vi "ConvertDesiredRefreshRatioPerReactor.vi"(0 "Desired Refresh Ratio":dbl, 2 "Reactor":i64 min=0 max=7) -> (1 "Required Number of Pump Iterations":dbl)   [LabVIEW 2016]
uses:
  CurrentSwitchValues_GlobalVariable.vi
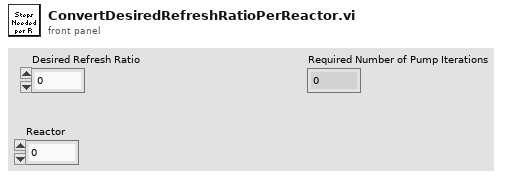
[diagram p1: front panel]
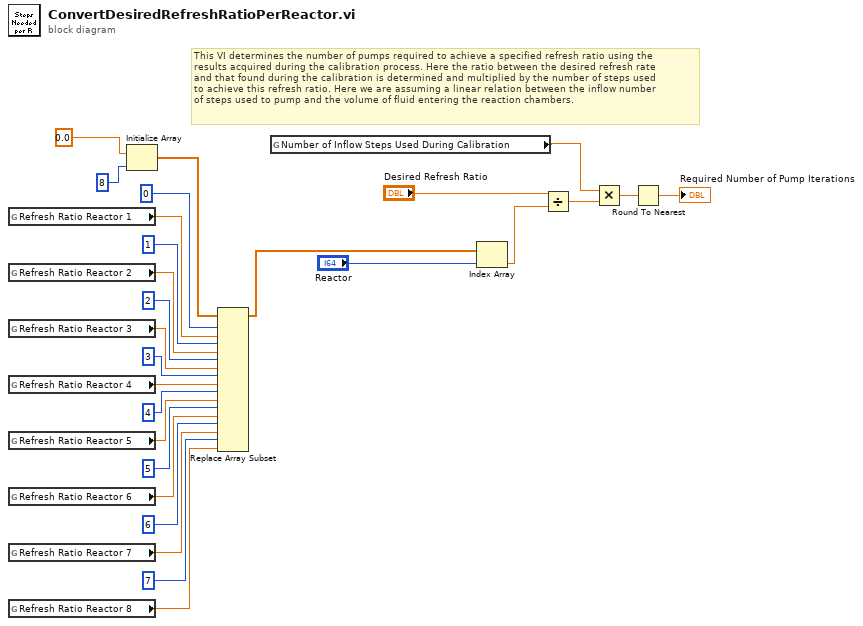
[diagram p0: block diagram]
diagram:
  # "This VI determines the number of pumps required to achieve a specified refresh ratio using the \nresults acquired during the calibration process. Here the ratio between the desired refresh rate \nand that found during the calibration is determined and multiplied by the number of steps used\nto achieve this refresh ratio. Here we are assuming a linear relation between the inflow number \nof steps used to pump and the volume of fluid entering the reaction chambers."
  n1 = global read "CurrentSwitchValues_GlobalVariable.vi" "Refresh Ratio Reactor 1"() -> (w16:dbl)
  n2 = global read "CurrentSwitchValues_GlobalVariable.vi" "Refresh Ratio Reactor 2"() -> (w15:dbl)
  n3 = global read "CurrentSwitchValues_GlobalVariable.vi" "Refresh Ratio Reactor 3"() -> (w14:dbl)
  n4 = global read "CurrentSwitchValues_GlobalVariable.vi" "Refresh Ratio Reactor 4"() -> (w13:dbl)
  n5 = global read "CurrentSwitchValues_GlobalVariable.vi" "Refresh Ratio Reactor 5"() -> (w12:dbl)
  n6 = global read "CurrentSwitchValues_GlobalVariable.vi" "Refresh Ratio Reactor 6"() -> (w11:dbl)
  n7 = global read "CurrentSwitchValues_GlobalVariable.vi" "Refresh Ratio Reactor 7"() -> (w10:dbl)
  n8 = global read "CurrentSwitchValues_GlobalVariable.vi" "Refresh Ratio Reactor 8"() -> (w9:dbl)
  n9 = Initialize Array(0.0, 8) -> (w17:dbl[])
  n10 = Replace Array Subset(array=w17, new element #1=w16, index #1=0, new element #2=w15, index #2=1, new element #3=w14, index #3=2, new element #4=w13, index #4=3, new element #5=w12, index #5=4, new element #6=w11, index #6=5, new element #7=w10, index #7=6, new element #8=w9, index #8=7) -> (w8:dbl[])
  n11 = global read "CurrentSwitchValues_GlobalVariable.vi" "Number of Inflow Steps Used During Calibration"() -> (w21:dbl)
  n12 = Index Array(array=w8, index="Reactor") -> (element=w23:dbl)
  n13 = Divide(x="Desired Refresh Ratio", y=w23) -> (x/y=w26:dbl)
  n14 = Multiply(x=w21, y=w26) -> (x*y=w25:dbl)
  n15 = Round To Nearest(number=w25) -> (nearest integer value=→"Required Number of Pump Iterations":dbl)
